vi "CalcVectorsold.vi"(6 "In/out":dbl, 9 "Up/down":dbl, 10 "Shoulder Degrees":dbl, 11 "Elbow Degrees":dbl) -> (2 "Shoulder Power":dbl, 3 "Elbow power":dbl)   [LabVIEW 2018]
panel:
  out "B Up-Down":dbl
  out "C-up/down":dbl
  out "B":dbl
  out "C":dbl
  out "Sin(a)":dbl
  out "Theta a":dbl
  out "sin(b)":dbl
  out "sin(c)":dbl
  out "Theta C":dbl
  out "Theta b":dbl
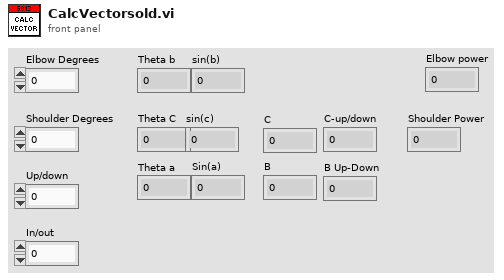
[diagram p1: front panel]
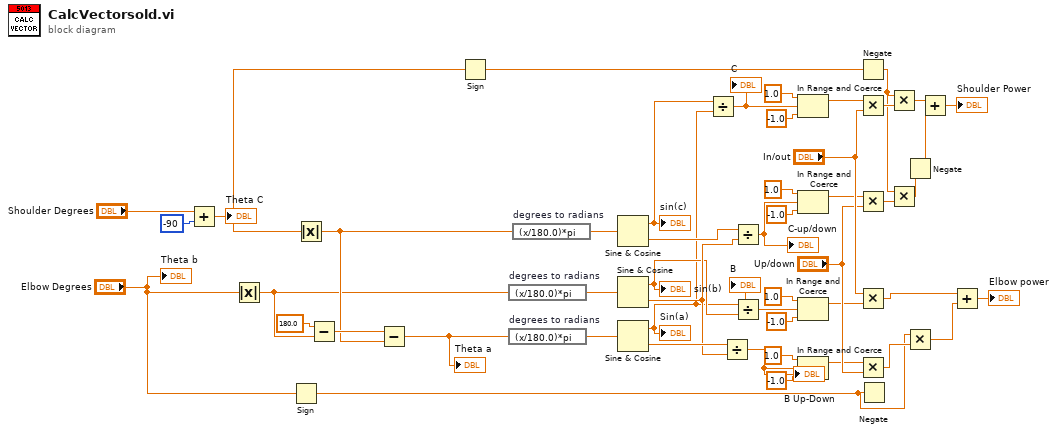
[diagram p0: block diagram]
diagram:
  n1 = Add(x="Shoulder Degrees", y=-90) -> (x+y=w37:dbl)
  "Theta C" <- w37
  n2 = Absolute Value(x="Elbow Degrees") -> (abs(x)=w35:dbl)
  n3 = Sign(1:"Elbow Degrees") -> (0:w9:dbl)
  n4 = Absolute Value(x=w37) -> (abs(x)=w36:dbl)
  n5 = Subtract(x=180.0, y=w35) -> (x-y=w38:dbl)
  n6 = Subtract(x=w38, y=w36) -> (x-y=w33:dbl)
  "Theta a" <- w33
  n7 = Sign(1:w37) -> (0:w8:dbl)
  n8 = expression code="(x/180.0)*pi" "degrees to radians"(w35) -> (w44:dbl)
  n9 = expression code="(x/180.0)*pi" "degrees to radians"(w33) -> (w34:dbl)
  n10 = expression code="(x/180.0)*pi" "degrees to radians"(w36) -> (w47:dbl)
  n11 = Sine & Cosine(0:w47) -> (1:w1:dbl, 2:w6:dbl)
  "sin(c)" <- w1
  n12 = Sine & Cosine(0:w44) -> (1:w3:dbl, 2:w5:dbl)
  "sin(b)" <- w3
  n13 = Sine & Cosine(0:w34) -> (1:w2:dbl, 2:w24:dbl)
  "Sin(a)" <- w2
  n14 = Divide(x=w1, y=w2) -> (x/y=w42:dbl)
  "C" <- w42
  n15 = Divide(x=w24, y=w5) -> (x/y=w29:dbl)
  "B Up-Down" <- w29
  n16 = Divide(x=w6, y=w5) -> (x/y=w31:dbl)
  "C-up/down" <- w31
  n17 = Divide(x=w2, y=w3) -> (x/y=w41:dbl)
  "B" <- w41
  n18 = In Range and Coerce(upper limit=1.0, x=w42, lower limit=-1.0) -> (coerced(x)=w23:dbl)  [unwired: 1 out]
  n19 = In Range and Coerce(upper limit=1.0, x=w31, lower limit=-1.0) -> (coerced(x)=w20:dbl)  [unwired: 1 out]
  n20 = In Range and Coerce(upper limit=1.0, x=w41, lower limit=-1.0) -> (coerced(x)=w17:dbl)  [unwired: 1 out]
  n21 = In Range and Coerce(upper limit=1.0, x=w29, lower limit=-1.0) -> (coerced(x)=w14:dbl)  [unwired: 1 out]
  n22 = Negate(x=w8) -> (-x=w7:dbl)
  n23 = Multiply(x=w23, y="In/out") -> (x*y=w49:dbl)
  n24 = Multiply(x=w20, y="Up/down") -> (x*y=w25:dbl)
  n25 = Multiply(x="In/out", y=w17) -> (x*y=w48:dbl)
  n26 = Multiply(x=w14, y="Up/down") -> (x*y=w27:dbl)
  n27 = Negate(x=w9) -> ()  [unwired: 1 out]
  n28 = Multiply(x=w7, y=w49) -> (x*y=w40:dbl)
  n29 = Multiply(x=w7, y=w25) -> (x*y=w10:dbl)
  n30 = Negate(x=w10) -> (-x=w4:dbl)
  n31 = Multiply(x=w9, y=w27) -> (x*y=w11:dbl)
  n32 = Add(x=w40, y=w4) -> (x+y=→"Shoulder Power":dbl)
  n33 = Add(x=w48, y=w11) -> (x+y=→"Elbow power":dbl)
  "Theta b" <- "Elbow Degrees"
